vi "NMRFMTCP6test.vi"() -> ()   [LabVIEW 2013]
uses:
  <vilib>/Analysis/2dsp.llb/Power Spectrum (DBL).vi
  kleinjan/MKS/Global - Pressure & Flow.vi
  <vilib>/Analysis/NI_AALBase.lvlib
  <vilib>/Analysis/NI_AALPro.lvlib
panel:
  out "Python OK":bool=TRUE
  out "Polarization":sgl=36.423462 format="%.3f"
  out "+3.3V OK":bool=TRUE
  out "Qsub OK":bool
  out "standard error":string
  out "standard output":string
  out "return code":i32
  out "initphase":dbl=2.566 format="%#_13g"
  out "inittune":dbl=1.9 format="%#_13g"
  in  "Save Tune":bool
  in  "Tune?":bool
  out "Date / Time":string="1/31/2018 1:50:59 PM"
  in  "Stop Run":bool=TRUE
  out "He readback":bool=TRUE
  in  "Prompt?":bool
  out "He temp (K)":sgl=2.13326 format="%.3f"
  out "He press (torr)":sgl=33.89 format="%.3f"
  in  "NMR Channel Select":string(combo)="Tune2.csv"
  out "Color Box":u32(colorbox)=16775210
  out "Measurement":enum16{"TEQ", "POL", "QCV"}(ring)
  in  "VME IP Address":string="192.168.0.4"
  out "FFT Vrms":dbl[](graph)=[0.06867481296758104, 0.06857457198498951, 0.06260490220323817, 0.04579893096764441, 0.03459193119021722, 0.024334506004456635, 0.01699939743179473, 0.011320507920014591, 0.00738818639942318, 0.004922329269476129, 0.0032005220838690783, 0.002399742088009097, 0.0017369883972344268, 0.001462379050983699, 0.0012180378187000385, 0.0009973302434478017, 0.0008651345258721481, 0.0006297489865595406, 0.0005526001513740785, 0.00037281048607525053, 0.00030391613013233313, 0.00020982577489229117, 0.00011097556197799909, 9.224206231092217e-05, 6.542017012320741e-05, 9.304661554256529e-05, 5.856346737504307e-05, 7.273895027450311e-05, 7.459248680725348e-05, 2.878408363596768e-05, 6.035598396088183e-05, 1.2803091312800212e-05, 3.242558212250914e-05, 2.6299059518835237e-05, 2.8629288070241252e-05, 5.5072971721899855e-05, 6.084837494592859e-06, 1.8134519288074238e-05, 9.669082428092558e-06, 1.0358869367749575e-05, 1.018912080523636e-05, 8.60594191940927e-06, 9.591448625769922e-06, 1.1220166852002886e-05, 6.88011593273858e-06, 1.1491109330674236e-05, 1.6694054808243664e-05, 1.0324476781176234e-06, 8.726383764090988e-06, 1.0009405679331725e-05, 6.983276809422243e-06, 1.0990654268439946e-05, 6.235393540925832e-06, 1.3028318573115987e-05, 8.212929592602332e-06, 7.620469710636132e-06, 1.3517970354642288e-05, 3.1360145539364084e-06, 1.0966864774965756e-05, 1.8371644041724748e-06, 1.4366548133168728e-05, 1.8995353004426356e-05, 1.261262728619325e-05, 1.1944444533945176e-05, 6.099138601232397e-06, 1.693319713220885e-05, 1.5290407351991908e-05, 1.554922736223277e-05, 1.1123224499577624e-05, 5.543972521096801e-07, 1.2984947025426147e-05, 1.8988972689681565e-05, 1.4206861079379492e-05, 2.1083207681653224e-05, 1.6007929951300866e-05, 2.7877039602988794e-05, 1.0482172647931049e-05, 1.8537108589101367e-05, 5.604028017532567e-06, 5.635675332586378e-06, 1.0245787700958885e-05, 3.285883828179235e-06, 8.512312116457392e-06, 1.4595660468423015e-05, 3.3757230764538894e-06, 1.1434598449200437e-05, 9.009063554776636e-06, 9.09203278507544e-06, 8.614121129346514e-06, 2.7065739961170123e-06, 6.030594935431283e-06, 1.1022840446923136e-05, 3.4608859994916356e-06, 1.1678562894888675e-05, 6.324112407218391e-06, 6.1924960014341965e-06, 4.748606861354588e-06, 2.768720553267083e-06, 5.808055347668398e-06, 4.95687957388527e-06, 4.552721418323117e-06, 4.868943846160484e-06, 3.4341407516096863e-06, 5.5974628740544295e-06, 4.241367499491773e-06, 6.586740589704174e-06, 4.024549450977876e-06, 5.122947155766902e-06, 3.9773543460348965e-06, 6.5077684618683735e-06, 4.010278671524191e-06, 4.121194802615129e-06, 3.282257530443253e-06, 2.5860963363552985e-06, 9.189431625458063e-06, 7.099592745613212e-06, 5.333822391148828e-06, 5.943090011187765e-06, 4.309063888021288e-06, 3.5031630262908657e-06, 1.96922856062359e-06, 4.6071849490317016e-07, 6.351051902186674e-06, 4.122666103856541e-06, 6.469252923693759e-06, 1.8226265223917853e-06, 8.244885041838854e-06, 1.6345124528207519e-06, 4.601201303647493e-06, 8.496993206144022e-06, 3.5355491948303763e-06, 7.895706171681286e-06, 5.645936982007796e-06, 3.7385657954831592e-06, 8.727751684292659e-06, 4.869286516414961e-06, 7.81165746958526e-06, 4.667304716818145e-06, 5.081172661891545e-06, 6.686448783162224e-06, 4.00495839673786e-06, 1.1485451036657622e-05, 2.6838919673161818e-06, 1.1144088742135484e-05, 4.668724848017115e-06, 4.9955017370136556e-06, 1.6524892105897692e-06, 1.144022174967641e-06, 6.6432326246144885e-06, 4.840482493249558e-06, 1.2421741122621969e-05, 3.74322163703047e-06, 8.703797353115438e-06, 4.388068688090438e-06, 2.9175286376936667e-06, 3.3209910498661074e-06, 5.7511551959757365e-06, 3.0725434377290935e-06, 2.2189801998406774e-06, 6.073062826056792e-06, 5.407884797516531e-06, 3.323217205604381e-06, 8.478322260705957e-06, 2.4801854003522035e-06, 8.379497453356208e-06, 1.7697452972367595e-06, 7.3317561052701325e-06, 4.226726258326851e-06, 4.623660588236943e-06, 7.655373604817283e-06, 9.087980261541697e-07, 6.199940244089063e-06, 5.437223520954798e-07, 4.066597652669098e-06, 3.6919111735151345e-06, 4.291749516194073e-06, 5.610961626882009e-06, 2.5547763024940687e-06, 2.498718509567958e-06, 1.227414154389083e-05, 6.558351876350384e-06, 2.609450378482884e-06, 7.39055217848152e-06, 2.5707380987801505e-06, 5.649112772736493e-06, 5.415988675717733e-06, 5.239708070750125e-06, 2.7406394221776962e-06, 8.059224052285553e-06, 3.981707950065012e-06, 2.2827311665321965e-07, 4.762940780814428e-06, 2.2866533297097247e-06, 2.1480718211679797e-06, 8.711481544735441e-06, 4.8420425852430605e-06, 1.082893263992563e-06, 5.394159492985945e-06, 4.286252813980868e-06, 7.453130120166451e-06, 1.6277649462102944e-06, 1.6277649462102944e-06, 7.453130120166451e-06, 4.286252813980868e-06, 5.394159492985945e-06, 1.082893263992563e-06, 4.8420425852430605e-06, 8.711481544735441e-06, 2.1480718211679797e-06, 2.2866533297097247e-06, 4.762940780814428e-06, 2.2827311665321965e-07, 3.981707950065012e-06, 8.059224052285553e-06, 2.7406394221776962e-06, 5.239708070750125e-06, 5.415988675717733e-06, 5.649112772736493e-06, 2.5707380987801505e-06, 7.39055217848152e-06, 2.609450378482884e-06, 6.558351876350384e-06, 1.227414154389083e-05, 2.498718509567958e-06, 2.5547763024940687e-06, 5.610961626882009e-06, 4.291749516194073e-06, 3.6919111735151345e-06, 4.066597652669098e-06, 5.437223520954798e-07, 6.199940244089063e-06, 9.087980261541697e-07, 7.655373604817283e-06, 4.623660588236943e-06, 4.226726258326851e-06, 7.3317561052701325e-06, 1.7697452972367595e-06, 8.379497453356208e-06, 2.4801854003522035e-06, 8.478322260705957e-06, 3.323217205604381e-06, 5.407884797516531e-06, 6.073062826056792e-06, 2.2189801998406774e-06, 3.0725434377290935e-06, 5.7511551959757365e-06, 3.3209910498661074e-06, 2.9175286376936667e-06, 4.388068688090438e-06, 8.703797353115438e-06, 3.74322163703047e-06, 1.2421741122621969e-05, 4.840482493249558e-06, 6.6432326246144885e-06, 1.144022174967641e-06, 1.6524892105897692e-06, 4.9955017370136556e-06, 4.668724848017115e-06, 1.1144088742135484e-05, 2.6838919673161818e-06, 1.1485451036657622e-05, 4.00495839673786e-06, 6.686448783162224e-06, 5.081172661891545e-06, 4.667304716818145e-06, 7.81165746958526e-06, 4.869286516414961e-06, 8.727751684292659e-06, 3.7385657954831592e-06, 5.645936982007796e-06, 7.895706171681286e-06, 3.5355491948303763e-06, 8.496993206144022e-06, 4.601201303647493e-06, 1.6345124528207519e-06, 8.244885041838854e-06, 1.8226265223917853e-06, 6.469252923693759e-06, 4.122666103856541e-06, 6.351051902186674e-06, 4.6071849490317016e-07, 1.96922856062359e-06, 3.5031630262908657e-06, 4.309063888021288e-06, 5.943090011187765e-06, 5.333822391148828e-06, 7.099592745613212e-06, 9.189431625458063e-06, 2.5860963363552985e-06, 3.282257530443253e-06, 4.121194802615129e-06, 4.010278671524191e-06, 6.5077684618683735e-06, 3.9773543460348965e-06, 5.122947155766902e-06, 4.024549450977876e-06, 6.586740589704174e-06, 4.241367499491773e-06, 5.5974628740544295e-06, 3.4341407516096863e-06, 4.868943846160484e-06, 4.552721418323117e-06, 4.95687957388527e-06, 5.808055347668398e-06, 2.768720553267083e-06, 4.748606861354588e-06, 6.1924960014341965e-06, 6.324112407218391e-06, 1.1678562894888675e-05, 3.4608859994916356e-06, 1.1022840446923136e-05, 6.030594935431283e-06, 2.7065739961170123e-06, 8.614121129346514e-06, 9.09203278507544e-06, 9.009063554776636e-06, 1.1434598449200437e-05, 3.3757230764538894e-06, 1.4595660468423015e-05, 8.512312116457392e-06, 3.285883828179235e-06, 1.0245787700958885e-05, 5.635675332586378e-06, 5.604028017532567e-06, 1.8537108589101367e-05, 1.0482172647931049e-05, 2.7877039602988794e-05, 1.6007929951300866e-05, 2.1083207681653224e-05, 1.4206861079379492e-05, 1.8988972689681565e-05, 1.2984947025426147e-05, 5.543972521096801e-07, 1.1123224499577624e-05, 1.554922736223277e-05, 1.5290407351991908e-05, 1.693319713220885e-05, 6.099138601232397e-06, 1.1944444533945176e-05, 1.261262728619325e-05, 1.8995353004426356e-05, 1.4366548133168728e-05, 1.8371644041724748e-06, 1.0966864774965756e-05, 3.1360145539364084e-06, 1.3517970354642288e-05, 7.620469710636132e-06, 8.212929592602332e-06, 1.3028318573115987e-05, 6.235393540925832e-06, 1.0990654268439946e-05, 6.983276809422243e-06, 1.0009405679331725e-05, 8.726383764090988e-06, 1.0324476781176234e-06, 1.6694054808243664e-05, 1.1491109330674236e-05, 6.88011593273858e-06, 1.1220166852002886e-05, 9.591448625769922e-06, 8.60594191940927e-06, 1.018912080523636e-05, 1.0358869367749575e-05, 9.669082428092558e-06, 1.8134519288074238e-05, 6.084837494592859e-06, 5.5072971721899855e-05, 2.8629288070241252e-05, 2.6299059518835237e-05, 3.242558212250914e-05, 1.2803091312800212e-05, 6.035598396088183e-05, 2.878408363596768e-05, 7.459248680725348e-05, 7.273895027450311e-05, 5.856346737504307e-05, 9.304661554256529e-05, 6.542017012320741e-05, 9.224206231092217e-05, 0.00011097556197799909, 0.00020982577489229117, 0.00030391613013233313, 0.00037281048607525053, 0.0005526001513740785, 0.0006297489865595406, 0.0008651345258721481, 0.0009973302434478017, 0.0012180378187000385, 0.001462379050983699, 0.0017369883972344268, 0.002399742088009097, 0.0032005220838690783, 0.004922329269476129, 0.00738818639942318, 0.011320507920014591, 0.01699939743179473, 0.024334506004456635, 0.03459193119021722, 0.04579893096764441, 0.06260490220323817, 0.06857457198498951]
  out "Raw NMR Graph / Ave":cluster{dbl, "Step Width (MHz)":dbl, dbl[][]}(graph)={212.6, "Step Width (MHz)"=0.002, [[0.0092, 0.0092, 0.0092, 0.009, 0.0087, 0.0085, 0.0082, 0.0078, 0.0075, 0.0072, 0.0069, 0.0066, 0.0061, 0.006, 0.0058, 0.0055, 0.0052, 0.005, 0.0047, 0.0044, 0.0043, 0.0041, 0.0041, 0.0037, 0.0037, 0.0034, 0.0032, 0.0029, 0.0024, 0.0021, 0.0017, 0.0015, 0.0012, 0.0009, 0.0008, 0.0008, 0.0006, 0.0005, 0.0003, 0.0003, -0.0, -0.0002, -0.0005, -0.0006, -0.0009, -0.0011, -0.0014, -0.0017, -0.0018, -0.002, -0.0023, -0.0026, -0.0026, -0.0027, -0.0027, -0.0031, -0.0029, -0.0032, -0.0032, -0.0032, -0.0034, -0.0037, -0.0037, -0.0041, -0.0043, -0.0044, -0.0046, -0.0047, -0.0047, -0.0047, -0.0049, -0.0049, -0.005, -0.0049, -0.005, -0.0052, -0.0055, -0.0055, -0.0056, -0.0056, -0.0056, -0.0058, -0.006, -0.0061, -0.0061, -0.0063, -0.0063, -0.0064, -0.0064, -0.0064, -0.0064, -0.0063, -0.0061, -0.0061, -0.0061, -0.0061, -0.0061, -0.0061, -0.0061, -0.0061, -0.0063, -0.0063, -0.0061, -0.006, -0.006, -0.0056, -0.0053, -0.0052, -0.005, -0.0049, -0.0047, -0.0044, -0.0043, -0.0041, -0.0038, -0.0037, -0.0034, -0.0031, -0.0029, -0.0026, -0.0024, -0.0021, -0.0018, -0.0015, -0.0009, -0.0006, -0.0, 0.0003, 0.0009, 0.0015, 0.002, 0.0026, 0.0031, 0.0035, 0.0041, 0.0047, 0.0052, 0.0058, 0.0066, 0.0073, 0.0082, 0.0092, 0.0099, 0.011, 0.0119, 0.013, 0.014, 0.0151, 0.016, 0.0172, 0.0186, 0.0198, 0.0211, 0.0223, 0.0237, 0.0253, 0.027, 0.029, 0.0308, 0.033, 0.0352, 0.0378, 0.0403, 0.043, 0.0461, 0.049, 0.0522, 0.0555, 0.0592, 0.0632, 0.0674, 0.0722, 0.0771, 0.0822, 0.0879, 0.094, 0.1006, 0.1074, 0.1144, 0.1224, 0.1309, 0.1401, 0.1495, 0.1593, 0.1697, 0.1808, 0.1926, 0.2049, 0.2179, 0.231, 0.2454, 0.2605, 0.2759, 0.2922, 0.3087, 0.3261, 0.3433, 0.3609, 0.3789, 0.3967, 0.4143, 0.4314, 0.4485, 0.4655, 0.4817, 0.4973, 0.5115, 0.5258, 0.5396, 0.5525, 0.5644, 0.5754, 0.5856, 0.5954, 0.6039, 0.6108, 0.6163, 0.6203, 0.6227, 0.623, 0.6213, 0.6169, 0.6105, 0.6018, 0.591, 0.5774, 0.5606, 0.5417, 0.5203, 0.497, 0.4721, 0.4446, 0.4161, 0.3874, 0.3583, 0.3307, 0.304, 0.2774, 0.2525, 0.2295, 0.2086, 0.1898, 0.1729, 0.1567, 0.1419, 0.1286, 0.1166, 0.1057, 0.0954, 0.0859, 0.0775, 0.0699, 0.0627, 0.0562, 0.0502, 0.0447, 0.0397, 0.0352, 0.0308, 0.027, 0.0237, 0.0204, 0.0177, 0.015, 0.0125, 0.0104, 0.0082, 0.0066, 0.0047, 0.0031, 0.0015, -0.0, -0.0014, -0.0027, -0.0041, -0.0052, -0.0064, -0.0073, -0.0082, -0.0093, -0.0101, -0.0108, -0.0114, -0.0121, -0.0127, -0.0131, -0.0134, -0.0139, -0.0143, -0.0146, -0.0151, -0.0157, -0.0163, -0.0166, -0.0169, -0.0172, -0.0172, -0.0175, -0.0175, -0.0177, -0.0175, -0.0177, -0.0175, -0.0177, -0.0177, -0.0177, -0.0179, -0.0179, -0.0179, -0.0179, -0.0179, -0.0179, -0.0179, -0.0179, -0.0177, -0.0179, -0.0175, -0.0175, -0.0172, -0.0171, -0.0168, -0.0165, -0.0163, -0.016, -0.016, -0.0159, -0.0159, -0.0156, -0.0154, -0.0154, -0.0151, -0.0148, -0.0145, -0.0142, -0.0139, -0.0137, -0.0134, -0.0133, -0.013, -0.0128, -0.0125, -0.0124, -0.0119, -0.0117, -0.0114, -0.011, -0.0108, -0.0107, -0.0104, -0.0104, -0.0099, -0.0098, -0.0096, -0.0092, -0.0087, -0.0084, -0.0079, -0.0076, -0.0073, -0.007, -0.0069, -0.0067, -0.0064, -0.0061, -0.0058, -0.0056, -0.0052, -0.0049, -0.0046, -0.0043, -0.0038, -0.0037, -0.0031, -0.0027, -0.0023, -0.002, -0.0015, -0.0011, -0.0008, -0.0005, -0.0002, -0.0, 0.0002, 0.0006, 0.0008, 0.0012, 0.0015, 0.002, 0.0026, 0.0031, 0.0037, 0.004, 0.0044, 0.0047, 0.0049, 0.0053, 0.0056, 0.0058, 0.0061, 0.0063, 0.0066], [0.0, 0.0, 0.0, 0.0, 0.0, 0.0, 0.0, 0.0, 0.0, 0.0, 0.0, 0.0, 0.0, 0.0, 0.0, 0.0, 0.0, 0.0, 0.0, 0.0, 0.0, 0.0, 0.0, 0.0, 0.0, 0.0, 0.0, 0.0, 0.0, 0.0, 0.0, 0.0, 0.0, 0.0, 0.0, 0.0, 0.0, 0.0, 0.0, 0.0, 0.0, 0.0, 0.0, 0.0, 0.0, 0.0, 0.0, 0.0, 0.0, 0.0, 0.0, 0.0, 0.0, 0.0, 0.0, 0.0, 0.0, 0.0, 0.0, 0.0, 0.0, 0.0, 0.0, 0.0, 0.0, 0.0, 0.0, 0.0, 0.0, 0.0, 0.0, 0.0, 0.0, 0.0, 0.0, 0.0, 0.0, 0.0, 0.0, 0.0, 0.0, 0.0, 0.0, 0.0, 0.0, 0.0, 0.0, 0.0, 0.0, 0.0, 0.0, 0.0, 0.0, 0.0, 0.0, 0.0, 0.0, 0.0, 0.0, 0.0, 0.0, 0.0, 0.0, 0.0, 0.0, 0.0, 0.0, 0.0, 0.0, 0.0, 0.0, 0.0, 0.0, 0.0, 0.0, 0.0, 0.0, 0.0, 0.0, 0.0, 0.0, 0.0, 0.0, 0.0, 0.0, 0.0, 0.0, 0.0, 0.0, 0.0, 0.0, 0.0, 0.0, 0.0, 0.0, 0.0, 0.0, 0.0, 0.0, 0.0, 0.0, 0.0, 0.0, 0.0, 0.0, 0.0, 0.0, 0.0, 0.0, 0.0, 0.0, 0.0, 0.0, 0.0, 0.0, 0.0, 0.0, 0.0, 0.0, 0.0, 0.0, 0.0, 0.0, 0.0, 0.0, 0.0, 0.0, 0.0, 0.0, 0.0, 0.0, 0.0, 0.0, 0.0, 0.0, 0.0, 0.0, 0.0, 0.0, 0.0, 0.0, 0.0, 0.0, 0.0, 0.0, 0.0, 0.0, 0.0, 0.0, 0.0, 0.0, 0.0, 0.0, 0.0, 0.0, 0.0, 0.0, 0.0, 0.0, 0.0, 0.0, 0.0, 0.0, 0.0, 0.0, 0.0, 0.0, 0.0, 0.0, 0.0, 0.0, 0.0, 0.0, 0.0, 0.0, 0.0, 0.0, 0.0, 0.0, 0.0, 0.0, 0.0, 0.0, 0.0, 0.0, 0.0, 0.0, 0.0, 0.0, 0.0, 0.0, 0.0, 0.0, 0.0, 0.0, 0.0, 0.0, 0.0, 0.0, 0.0, 0.0, 0.0, 0.0, 0.0, 0.0, 0.0, 0.0, 0.0, 0.0, 0.0, 0.0, 0.0, 0.0, 0.0, 0.0, 0.0, 0.0, 0.0, 0.0, 0.0, 0.0, 0.0, 0.0, 0.0, 0.0, 0.0, 0.0, 0.0, 0.0, 0.0, 0.0, 0.0, 0.0, 0.0, 0.0, 0.0, 0.0, 0.0, 0.0, 0.0, 0.0, 0.0, 0.0, 0.0, 0.0, 0.0, 0.0, 0.0, 0.0, 0.0, 0.0, 0.0, 0.0, 0.0, 0.0, 0.0, 0.0, 0.0, 0.0, 0.0, 0.0, 0.0, 0.0, 0.0, 0.0, 0.0, 0.0, 0.0, 0.0, 0.0, 0.0, 0.0, 0.0, 0.0, 0.0, 0.0, 0.0, 0.0, 0.0, 0.0, 0.0, 0.0, 0.0, 0.0, 0.0, 0.0, 0.0, 0.0, 0.0, 0.0, 0.0, 0.0, 0.0, 0.0, 0.0, 0.0, 0.0, 0.0, 0.0, 0.0, 0.0, 0.0, 0.0, 0.0, 0.0, 0.0, 0.0, 0.0, 0.0, 0.0, 0.0, 0.0, 0.0, 0.0, 0.0, 0.0, 0.0, 0.0, 0.0, 0.0, 0.0, 0.0, 0.0, 0.0, 0.0, 0.0, 0.0, 0.0, 0.0, 0.0, 0.0, 0.0, 0.0, 0.0, 0.0, 0.0, 0.0, 0.0, 0.0, 0.0, 0.0, 0.0, 0.0, 0.0, 0.0, 0.0, 0.0, 0.0, 0.0, 0.0, 0.0, 0.0, 0.0, 0.0, 0.0, 0.0, 0.0, 0.0, 0.0, 0.0, 0.0], [0.0, 0.0, 0.0, 0.0, 0.0, 0.0, 0.0, 0.0, 0.0, 0.0, 0.0, 0.0, 0.0, 0.0, 0.0, 0.0, 0.0, 0.0, 0.0, 0.0, 0.0, 0.0, 0.0, 0.0, 0.0, 0.0, 0.0006, 0.0006, 0.0004, 0.0003, 0.0003, 0.0003, 0.0001, 0.0, -0.0001, -0.0001, -0.0001, -0.0001, -0.0001, -0.0002, -0.0002, -0.0002, -0.0003, -0.0003, -0.0003, -0.0002, -0.0003, -0.0002, -0.0002, -0.0001, -0.0002, -0.0002, -0.0002, -0.0002, -0.0002, -0.0003, -0.0003, -0.0002, -0.0002, -0.0001, -0.0002, -0.0001, -0.0001, -0.0001, -0.0001, -0.0001, 0.0001, 0.0001, 0.0002, 0.0003, 0.0004, 0.0005, 0.0005, 0.0006, 0.0007, 0.0007, 0.0007, 0.0008, 0.0008, 0.001, 0.0011, 0.0012, 0.0013, 0.0015, 0.0016, 0.0016, 0.0018, 0.0019, 0.0021, 0.0022, 0.0023, 0.0025, 0.0028, 0.0029, 0.0031, 0.0033, 0.0035, 0.0037, 0.0039, 0.0041, 0.0042, 0.0044, 0.0047, 0.005, 0.0053, 0.0056, 0.006, 0.0062, 0.0065, 0.0067, 0.0072, 0.0074, 0.0077, 0.0081, 0.0086, 0.009, 0.0093, 0.0099, 0.0103, 0.0108, 0.0112, 0.0116, 0.012, 0.0125, 0.0131, 0.0136, 0.0141, 0.0147, 0.0154, 0.016, 0.0166, 0.0173, 0.0179, 0.0186, 0.0193, 0.0201, 0.0208, 0.0217, 0.0226, 0.0235, 0.0244, 0.0254, 0.0263, 0.0272, 0.0283, 0.0293, 0.0305, 0.0316, 0.0328, 0.0341, 0.0355, 0.037, 0.0385, 0.0399, 0.0415, 0.0433, 0.0452, 0.0471, 0.0491, 0.0514, 0.0537, 0.0562, 0.0588, 0.0616, 0.0646, 0.0678, 0.0712, 0.0748, 0.0786, 0.0828, 0.0872, 0.092, 0.097, 0.1023, 0.108, 0.1141, 0.1208, 0.1275, 0.1347, 0.1427, 0.1512, 0.1606, 0.17, 0.1796, 0.1902, 0.2015, 0.2135, 0.2259, 0.2388, 0.2523, 0.2668, 0.282, 0.2974, 0.3138, 0.3302, 0.3475, 0.365, 0.3826, 0.4006, 0.4185, 0.4362, 0.4535, 0.4706, 0.4876, 0.504, 0.5195, 0.5338, 0.5482, 0.5621, 0.5751, 0.5871, 0.598, 0.6084, 0.6181, 0.6266, 0.6335, 0.639, 0.643, 0.6453, 0.6458, 0.6438, 0.6396, 0.6333, 0.6247, 0.614, 0.6005, 0.584, 0.565, 0.5435, 0.5202, 0.4953, 0.4677, 0.4392, 0.4106, 0.3814, 0.3539, 0.3271, 0.3006, 0.2759, 0.2529, 0.2321, 0.2135, 0.1966, 0.1805, 0.1657, 0.1524, 0.1404, 0.1295, 0.1191, 0.1095, 0.101, 0.0931, 0.0862, 0.0795, 0.0733, 0.068, 0.0629, 0.0585, 0.0542, 0.0505, 0.0471, 0.0439, 0.0411, 0.0383, 0.0358, 0.0335, 0.0313, 0.0293, 0.0274, 0.0257, 0.024, 0.0225, 0.0212, 0.0198, 0.0185, 0.0174, 0.0163, 0.0152, 0.0143, 0.0134, 0.0125, 0.0116, 0.0108, 0.0101, 0.0094, 0.0088, 0.0083, 0.0077, 0.0072, 0.0067, 0.0062, 0.0056, 0.0053, 0.0048, 0.0044, 0.004, 0.0037, 0.0035, 0.0033, 0.003, 0.0028, 0.0025, 0.0023, 0.002, 0.0018, 0.0016, 0.0015, 0.0013, 0.0012, 0.0011, 0.001, 0.0009, 0.0008, 0.0007, 0.0006, 0.0004, 0.0004, 0.0003, 0.0003, 0.0003, 0.0002, 0.0003, 0.0002, 0.0002, 0.0002, 0.0001, 0.0001, 0.0, -0.0, -0.0, -0.0, 0.0, 0.0, 0.0001, 0.0001, 0.0, 0.0001, -0.0001, -0.0001, -0.0001, -0.0002, -0.0001, -0.0, -0.0, 0.0, 0.0, 0.0001, 0.0, 0.0001, 0.0, -0.0, -0.0, -0.0001, -0.0, 0.0001, 0.0001, 0.0001, 0.0, 0.0001, 0.0001, -0.0, -0.0, -0.0001, -0.0, 0.0, 0.0, 0.0001, 0.0001, 0.0, 0.0, 0.0001, -0.0, -0.0, -0.0001, -0.0001, 0.0, 0.0, 0.0, 0.0, 0.0, 0.0, 0.0, 0.0, 0.0, 0.0, 0.0, 0.0, 0.0, 0.0, 0.0, 0.0, 0.0, 0.0, 0.0, 0.0, 0.0, 0.0, 0.0, 0.0, 0.0, 0.0]]}
  in  "R&S GPIB Addr (28)":refnum<visa-resource-name>="GPIB0::28::INSTR"
  out "Pedestal (V)":dbl=-0.005459583333333334 format="%_2g"
  in  "Open Global Panel":bool
  out "Peak center (MHz)":sgl=213.038 format="%.3f"
  out "Telnet error out":errorcluster
  out "+3.3V supply":dbl=3.279 format="%_4g"
  out "Temp (C)":dbl=28.0 format="%_4g"
  out "RF level OK":bool=TRUE
  out "Polarization %":sgl=36.423462 format="%.3e"
  out "# Good Spectra":i32=494
  out "Pedestal volts OK":bool=TRUE
  out "Sweep #":i32=1
  out "1st Sweep":bool
  out "ADC volts OK":bool=TRUE
  out "Peak Height Distribution":cluster{"Y":dbl[], "Y":dbl[]}[](graph)=[{"Y"=[1.4880254648797504, 1.4904694004799532, 1.492913336080156, 1.495357271680359, 1.4978012072805618, 1.5002451428807646, 1.5026890784809674, 1.5051330140811703, 1.5075769496813731, 1.510020885281576, 1.5124648208817788, 1.5149087564819816, 1.5173526920821847, 1.5197966276823875, 1.5222405632825904, 1.5246844988827932, 1.527128434482996, 1.529572370083199, 1.5320163056834017, 1.5344602412836046, 1.5369041768838074, 1.5393481124840103, 1.541792048084213, 1.544235983684416, 1.5466799192846188, 1.5491238548848218, 1.5515677904850247, 1.5540117260852275, 1.5564556616854304, 1.5588995972856332, 1.561343532885836, 1.563787468486039, 1.5662314040862417, 1.5686753396864446, 1.5711192752866474, 1.5735632108868502, 1.576007146487053, 1.5784510820872562, 1.580895017687459, 1.5833389532876618, 1.5857828888878647, 1.5882268244880675, 1.5906707600882704, 1.5931146956884732, 1.595558631288676, 1.5980025668888789, 1.6004465024890817, 1.6028904380892846, 1.6053343736894874, 1.6077783092896902, 1.6102222448898933, 1.6126661804900961, 1.615110116090299, 1.6175540516905018, 1.6199979872907047, 1.6224419228909075, 1.6248858584911103, 1.6273297940913132, 1.629773729691516, 1.6322176652917189, 1.6346616008919217, 1.6371055364921245, 1.6395494720923276, 1.6419934076925304, 1.6444373432927333, 1.6468812788929361, 1.649325214493139, 1.6517691500933418, 1.6542130856935446, 1.6566570212937475, 1.6591009568939503, 1.6615448924941532, 1.663988828094356, 1.6664327636945588, 1.6688766992947617, 1.6713206348949647, 1.6737645704951676, 1.6762085060953704, 1.6786524416955733, 1.681096377295776, 1.683540312895979, 1.6859842484961818, 1.6884281840963846, 1.6908721196965875, 1.6933160552967903, 1.6957599908969931, 1.698203926497196, 1.700647862097399, 1.7030917976976019, 1.7055357332978047, 1.7079796688980076, 1.7104236044982104, 1.7128675400984132, 1.715311475698616, 1.717755411298819, 1.7201993468990218, 1.7226432824992246, 1.7250872180994274, 1.7275311536996303, 1.7299750892998331], "Y"=[3.0, 0.0, 0.0, 2.0, 1.0, 1.0, 0.0, 0.0, 2.0, 0.0, 2.0, 1.0, 2.0, 4.0, 2.0, 2.0, 0.0, 2.0, 2.0, 1.0, 5.0, 6.0, 7.0, 4.0, 5.0, 7.0, 3.0, 5.0, 5.0, 4.0, 5.0, 4.0, 7.0, 14.0, 7.0, 9.0, 12.0, 12.0, 8.0, 3.0, 5.0, 7.0, 6.0, 7.0, 8.0, 11.0, 7.0, 15.0, 12.0, 15.0, 15.0, 11.0, 8.0, 6.0, 11.0, 5.0, 6.0, 11.0, 14.0, 5.0, 6.0, 12.0, 9.0, 9.0, 3.0, 8.0, 13.0, 5.0, 6.0, 4.0, 10.0, 3.0, 5.0, 2.0, 6.0, 4.0, 5.0, 1.0, 4.0, 6.0, 3.0, 2.0, 0.0, 3.0, 4.0, 2.0, 2.0, 0.0, 2.0, 0.0, 4.0, 1.0, 2.0, 2.0, 0.0, 0.0, 0.0, 1.0, 0.0, 1.0]}]
  out "S/N":dbl=34.03525335839496 format="%_3g"
  out "Polarization %":dbl=1.6080975834470894 format="%_4g"
  out "Pedestal Diff (V)":sgl=-0.008144166 format="%.4f"
  out "Peak amp (mV)":sgl=351.93738 format="%.4f"
  out "SMT error out":errorcluster
  out "Pol sdev":dbl=47.24799802468473 format="%.3f"
  # "E1039 NMR Panel"
  # "Results"
  # "A\nv\ne\nr\na\ng\ne\ns"
  # "S\nw\ne\ne\np"
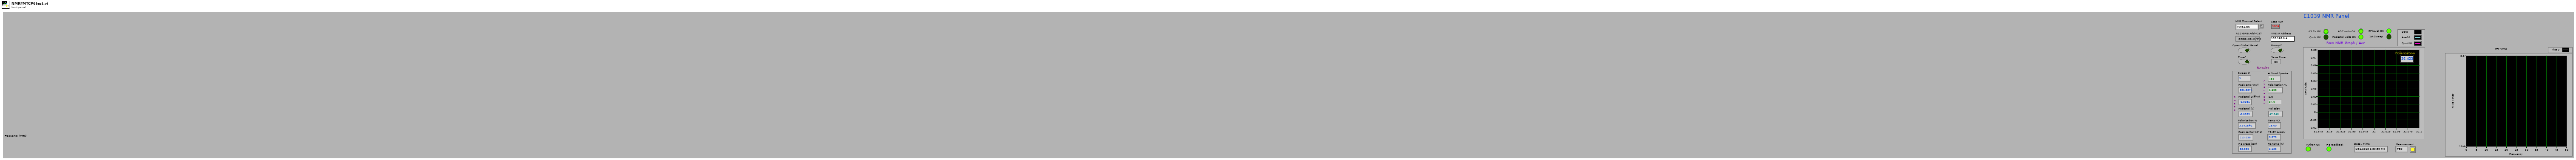
[diagram p1: front panel]
types:
  T1 = enum32{"Invalid", "Standard", "Closed", "Hidden", "Minimized", "Maximized"}
  T2 = enum32{"Bad", "Idle", "Run top level", "Running"}
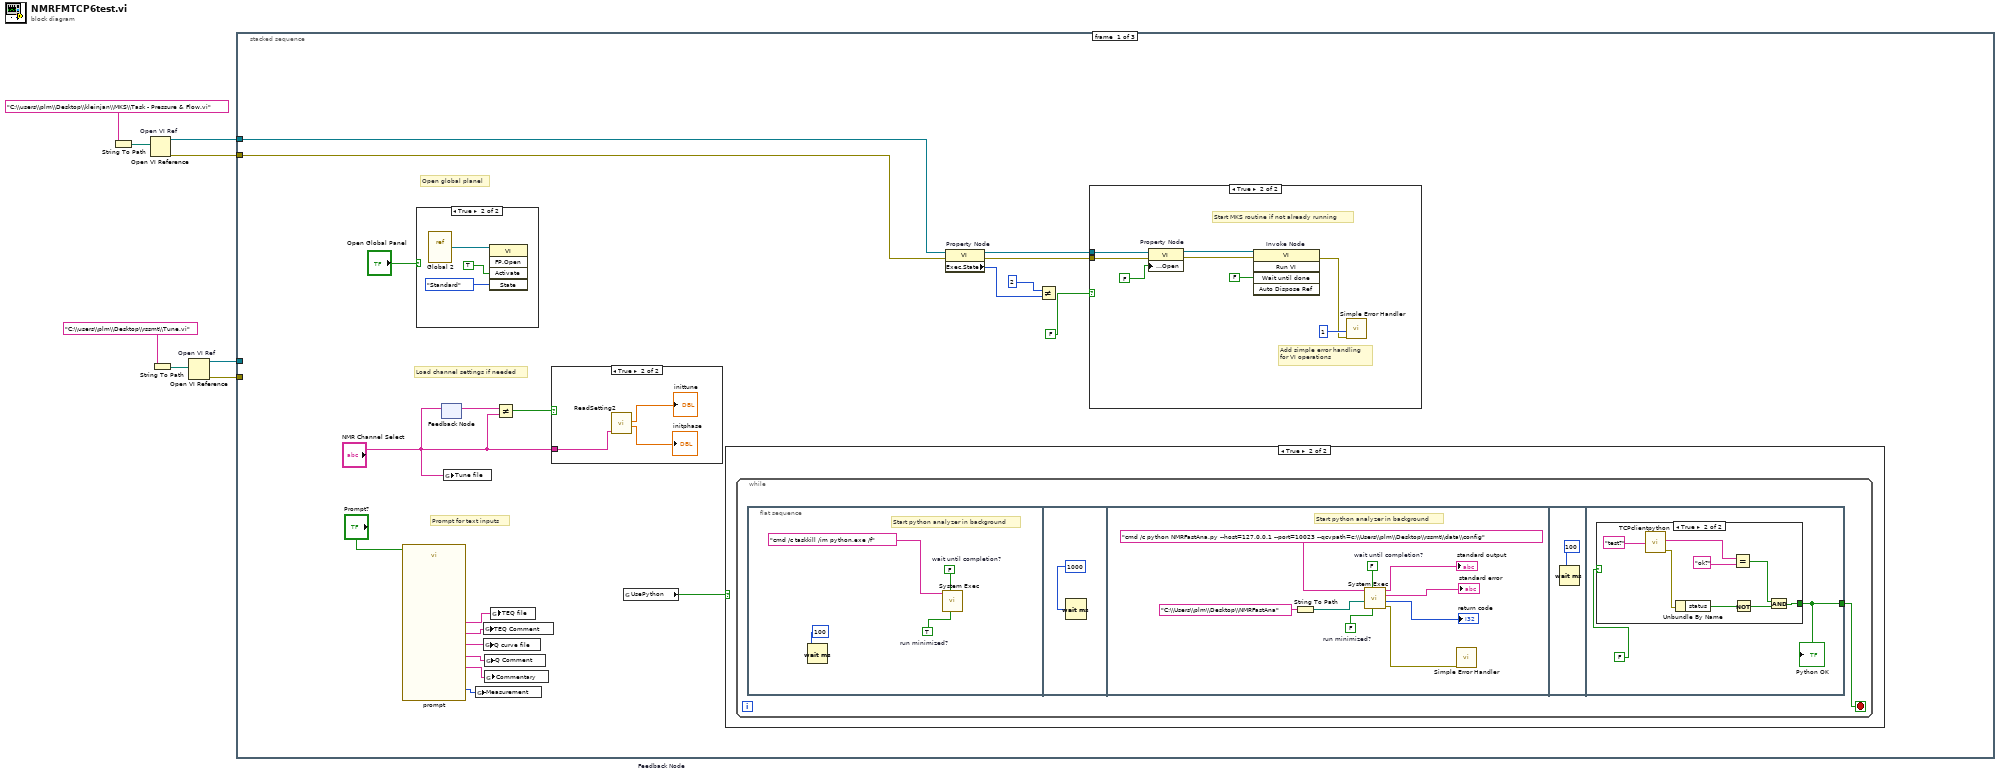
[diagram p0: block diagram]
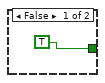
[diagram p3: hidden frame]
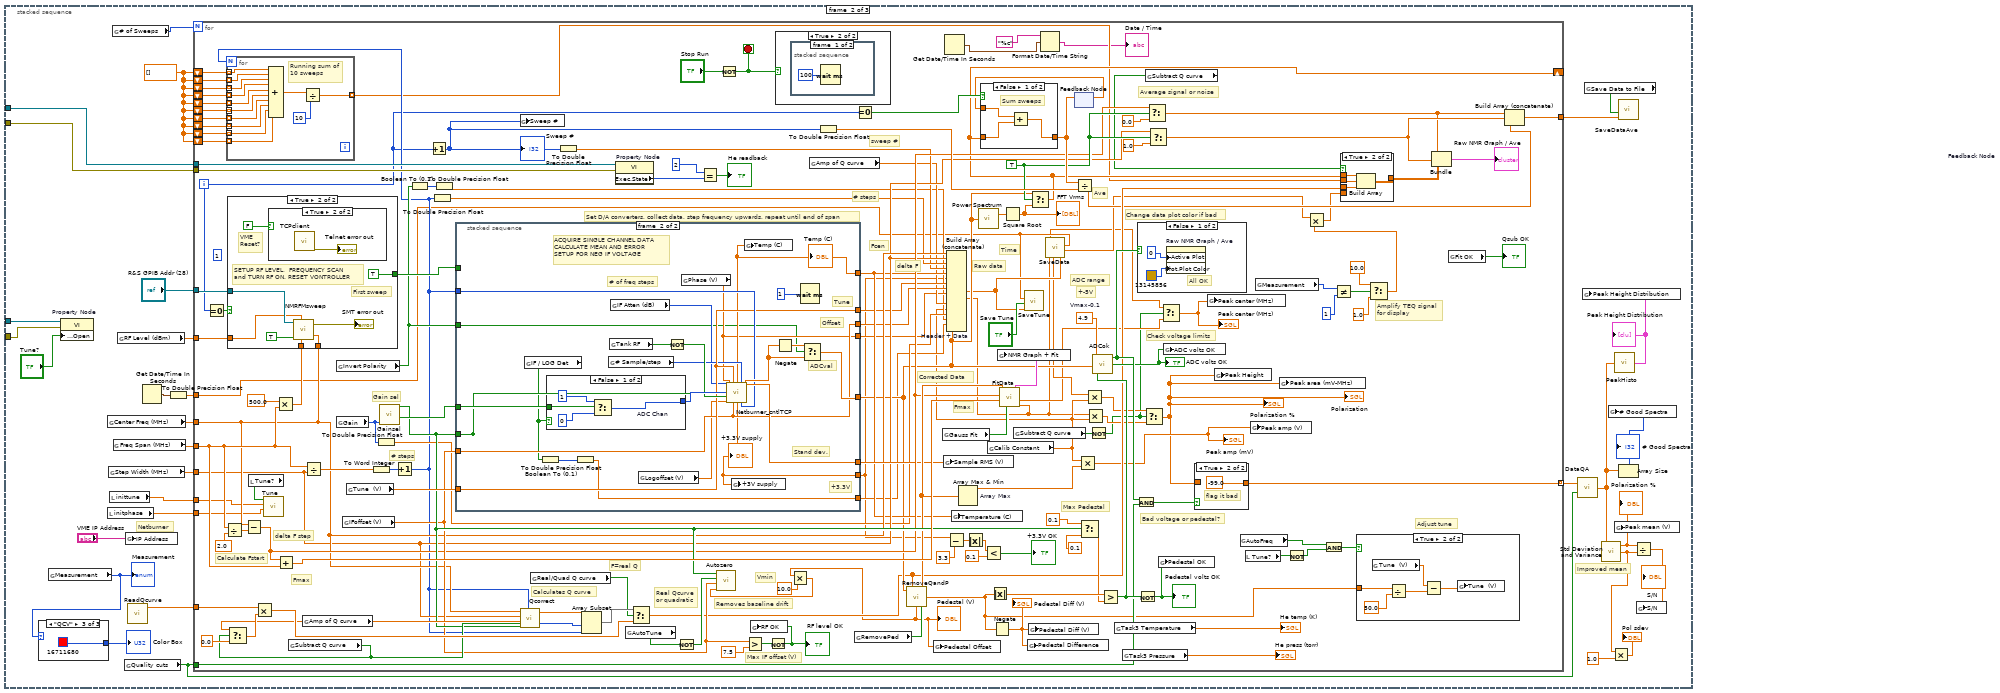
[diagram p7: hidden frame]
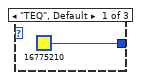
[diagram p8: hidden frame]
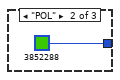
[diagram p9: hidden frame]
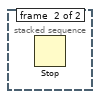
[diagram p12: hidden frame]
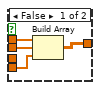
[diagram p13: hidden frame]
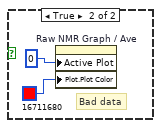
[diagram p15: hidden frame]
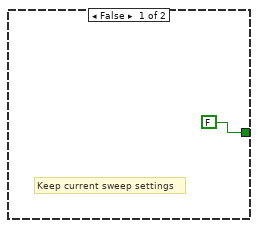
[diagram p17: hidden frame]
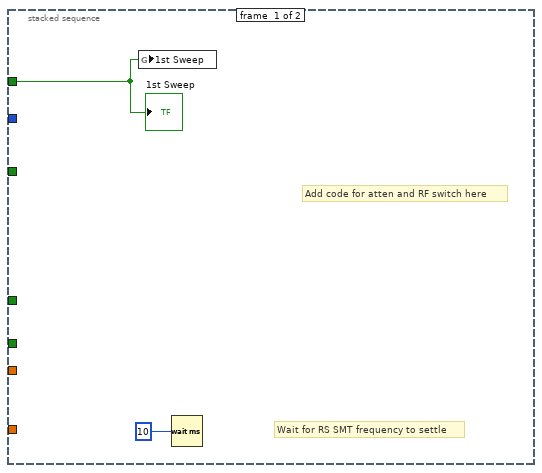
[diagram p19: hidden frame]
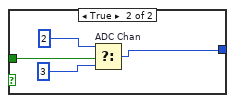
[diagram p20: hidden frame]
diagram:
  n1 = String To Path(string="C:\\users\\plm\\Desktop\\kleinjan\\MKS\\Task - Pressure & Flow.vi") -> (path=w8:path)
  n2 = Open VI Reference "Open VI Ref"(vi path=w8) -> (vi reference=w5:refnum<vi>, error out=w6:errorcluster)  [unwired: 5 in]
  n3 = String To Path(string="C:\\users\\plm\\Desktop\\rssmt\\Tune.vi") -> (path=w4:path)
  n4 = Open VI Reference "Open VI Ref"(vi path=w4) -> (vi reference=w2:refnum<vi>, error out=w1:errorcluster)  [unwired: 5 in]
  n5 = stacked-sequence {
    tunnel: w5 -> [w12 w76 w337]
    tunnel: w6 -> [w11 w75 w336]
    tunnel: w2 -> [_ w69 _]
    tunnel: w1 -> [_ w73 _]
    frame #0 {
      # "Prompt for text inputs"
      # "Load channel settings if needed"
      # "Open global planel"
      n6 = call "prompt.vi"("Enable"="Prompt?") -> ("Measurement"=w25:enum16{"TEQ", "POL", "QCV"}, "Run comment"=w24:string, "Q curve comment"=w23:string, "Q curve file"=w22:string, "TE Comment"=w21:string, "TE peak file"=w20:string)  [unwired: 11 in, 2 out]
      n7 = case shown="True" "Open Global Panel" {
        frame False {
        }
        frame True {
          n8 = vi-ref "Global 2.vi"() -> (w68:refnum<vi>)
          n9 = invoke class="VI" method="FP.Open"(reference=w68, "Activate"=TRUE, "State"=T1."Standard") -> ()  [unwired: 2 in, 5 out]
        }
      }
      n10 = feedback #1 "Feedback Node"() -> (w19:string)  [unwired: 1 in]
      n11 = feedback-in #1("NMR Channel Select") -> ()
      n12 = global write "Global 2.vi" "Tune file"("NMR Channel Select") -> ()
      n13 = global write "Global 2.vi" "Measurement"(w25) -> ()
      n14 = global write "Global 2.vi" "TEQ Comment"(w21) -> ()
      n15 = global write "Global 2.vi" "Q curve file"(w22) -> ()
      n16 = global write "Global 2.vi" "Q Comment"(w23) -> ()
      n17 = global write "Global 2.vi" "Commentary"(w24) -> ()
      n18 = global write "Global 2.vi" "TEQ file"(w20) -> ()
      n19 = Not Equal?(x=w19, y="NMR Channel Select") -> (x != y?=w18:bool)
      n20 = case shown="True" w18 {
        tunnel: "NMR Channel Select" -> [_ w65]
        frame False {
        }
        frame True {
          n21 = call "ReadSetting2.vi"("Data Filename"=w65) -> ("Phase"=→"initphase":dbl, "Tune"=→"inittune":dbl)  [unwired: 1 out]
        }
      }
      n22 = global read "Global 2.vi" "UsePython"() -> (w9:bool)
      n23 = case shown="True" w9 {
        frame False {
        }
        frame True {
          n24 = while {
            stop <- w28 stop-if-true
            n25 = flat-sequence {
              tunnel: [w45] -> w28
              frame #0 {
                w29 = TRUE  # run minimized?
                w30 = FALSE  # wait until completion?
                # "Start python analyzer in background"
                n26 = Wait (ms)(milliseconds to wait=100) -> ()  [unwired: 1 out]
                n27 = call <vilib>:"System Exec.vi"("run minimized? (F)"=w29, "wait until completion? (T)"=w30, "command line"="cmd /c taskkill /im python.exe /f") -> ()  [unwired: 5 in, 4 out]
              }
              frame #1 {
                n28 = Wait (ms)(milliseconds to wait=1000) -> ()  [unwired: 1 out]
              }
              frame #2 {
                w40 = FALSE  # run minimized?
                w41 = FALSE  # wait until completion?
                # "Start python analyzer in background"
                n29 = String To Path(string="C:\\Users\\plm\\Desktop\\NMRFastAna") -> (path=w35:path)
                n30 = call <vilib>:"System Exec.vi"("run minimized? (F)"=w40, "wait until completion? (T)"=w41, "working directory"=w35, "command line"="cmd /c python NMRFastAna.py --host=127.0.0.1 --port=10023 --qcvpath=c:\\Users\\plm\\Desktop\\rssmt\\data\\config") -> ("error out"=w36:errorcluster, "return code"=→"return code":i32, "standard error"=→"standard error":string, "standard output"=→"standard output":string)  [unwired: 4 in]
                n31 = call <vilib>:"Simple Error Handler.vi"("error in (no error)"=w36) -> ()  [unwired: 1 in, 8 out]
              }
              frame #3 {
                n32 = Wait (ms)(milliseconds to wait=100) -> ()  [unwired: 1 out]
              }
              frame #4 {
                n33 = case shown="True" FALSE {
                  tunnel: [TRUE w50] -> w45
                  frame False {
                  }
                  frame True {
                    n34 = call "TCPclientpython.vi"("Input Command"="test?") -> ("Telnet error"=w48:errorcluster, "Command and Results"=w53:string)  [unwired: 4 in, 1 out]
                    n35 = Unbundle By Name(w48) -> ("status"=w47:bool)
                    n36 = Equal?(x=w53, y="ok?") -> (x = y?=w51:bool)
                    n37 = Not(x=w47) -> (.not. x?=w49:bool)
                    n38 = And(x=w51, y=w49) -> (x .and. y?=w50:bool)
                  }
                }
                "Python OK" <- w45
              }
            }
          }
        }
      }
      n39 = property on="Property Node" class="VI"(reference=w12, error in=w11) -> (reference out=w14:refnum<vi>, error out=w13:errorcluster, "Exec.State"=w15:T2)
      n40 = Not Equal?(x=2, y=w15) -> ()  [unwired: 1 out]
      n41 = case shown="True" FALSE {
        tunnel: w14 -> [_ w59]
        tunnel: w13 -> [_ w58]
        frame False {
        }
        frame True {
          # "Start MKS routine if not already running"
          # "Add simple error handling\nfor VI operations"
          n42 = property on="Property Node" class="VI"(reference=w59, error in=w58, "Front Panel Window:Open"=FALSE ("Front Panel.Open")) -> (reference out=w57:refnum<vi>, error out=w56:errorcluster)
          n43 = invoke on="Invoke Node" class="VI" method="Run VI"(reference=w57, error in=w56, "Wait until done"=FALSE) -> (error out=w60:errorcluster)  [unwired: 2 in, 4 out]
          n44 = call <vilib>:"Simple Error Handler.vi"("type of dialog (OK msg:1)"=1, "error in (no error)"=w60) -> ()  [unwired: 3 in, 5 out]
        }
      }
    }
    frame #1 {
      w74 = dbl[] []
      # "Netburner"
      # "Improved mean"
      n45 = global read "Global 2.vi" "Measurement"() -> (w78:enum16{"TEQ", "POL", "QCV"})
      "Measurement" <- w78
      n46 = case shown="\"QCV\"" w78 {
        tunnel: [u32 16775210 ("Color Box 2") u32 3852288 ("Color Box 2") u32 16711680 ("Color Box 2")] -> w77
        frame "TEQ", Default {
        }
        frame "POL" {
        }
        frame "QCV" {
        }
      }
      "Color Box" <- w77
      n47 = property on="Property Node" class="VI"(reference=w69, error in=w73, "Front Panel Window:Open"="Tune?") -> ()  [unwired: 2 out]
      n48 = global read "Global 2.vi" "Center Freq (MHz)"() -> (w95:dbl)
      n49 = local read "initphase"() -> (w70:dbl)
      n50 = global read "Global 2.vi" "Step Width (MHz)"() -> (w93:dbl)
      n51 = local read "inittune"() -> (w71:dbl)
      n52 = global read "Global 2.vi" "# of Sweeps"() -> (w97:i32)
      n53 = global read "Global 2.vi" "Freq Span (MHz)"() -> (w94:dbl)
      n54 = global read "Global 2.vi" "RF Level (dBm)"() -> (w96:dbl)
      n55 = global read "Global 2.vi" "Quality cuts"() -> (w92:bool)
      n56 = global write "Global 2.vi" "IP Address"("VME IP Address") -> ()
      n57 = call "ReadQcurve.vi"() -> ("Array"=w83:dbl[])  [unwired: 2 in]
      n58 = Get Date/Time In Seconds() -> (seconds since 1Jan1904=w98:timestamp)
      n59 = To Double Precision Float(number=w98) -> (double precision float=w84:dbl)
      n60 = for {
        N: w97 -> [_]
        tunnel: [w247] -> w100 mode=indexing
        tunnel: w92 -> [w216]
        tunnel: w95 -> [w191]
        tunnel: w94 -> [w203]
        tunnel: w93 -> [w190]
        tunnel: "R&S GPIB Addr (28)" -> [w244]
        tunnel: w96 -> [w243]
        tunnel: w84 -> [w139]
        tunnel: w83 -> [w236]
        tunnel: [w206] -> w86
        tunnel: w76 -> [w169]
        tunnel: w75 -> [w168]
        shift-right: [w161] -> _
        shift-left: w74 -> [w160]
        shift-left: w74 -> [w151]
        shift-left: w74 -> [w159]
        shift-left: w74 -> [w158]
        shift-left: w74 -> [w157]
        shift-left: w74 -> [w156]
        shift-left: w74 -> [w155]
        shift-left: w74 -> [w154]
        shift-left: w74 -> [w153]
        shift-left: w74 -> [w152]
        tunnel: w71 -> [w143]
        tunnel: w70 -> [w142]
        i -> [w149]
        stop <- w141 stop-if-true
        (unwired) 1
        w196 = TRUE
        w211 = 4.9  # Vmax-0.1
        # "Amplify TEQ signal\nfor display"
        # "Adjust tune"
        # "Average signal or noise"
        # "Check voltage limits"
        # "Ave"
        # "Max Pedestal"
        # "Gain sel"
        # "F=real Q"
        # "Real Qcurve\nor quadratic"
        # "+-5V"
        # "Change data plot color if bad"
        # "Max IF offset (V)"
        # "Fmax"
        # "Fmax"
        # "Time"
        # "Vmin"
        # "Raw data"
        # "Corrected Data"
        # "Fcen"
        # "delta F"
        # "# steps"
        # "ADC range"
        # "sweep #"
        # "Set D/A converters, collect data, step frequency upwards, repeat until end of span"
        # "Calculates Q curve"
        # "Removes baseline drift"
        # "Bad voltage or pedestal?"
        # "# steps"
        # "Calculate Fstart"
        # "delta F step"
        n61 = Equal To 0?(x=w149) -> (x = 0?=w249:bool)
        n62 = Divide(x=w203, y=sgl 2.0) -> (x/y=w253:dbl)
        n63 = Subtract(x=w191, y=w253) -> (x-y=w194:dbl)
        n64 = local read "Tune?"() -> (w120:bool)
        n65 = call "Tune.vi"("Init Phase V"=w142, "Init Tune V"=w143, "Tune"=w120) -> ()  [unwired: 9 in]
        n66 = Multiply(x=500.0, y=w203) -> (x*y=w202:dbl)
        n67 = case shown="True" w249 {
          tunnel: w191 -> [_ w300]
          tunnel: w202 -> [_ w301]
          tunnel: [FALSE TRUE] -> w248
          tunnel: w244 -> [_ w297]
          tunnel: w243 -> [_ w296]
          frame False {
            # "Keep current sweep settings"
          }
          frame True {
            # "VME\nReset?"
            # "First sweep"
            # "SETUP RF LEVEL,  FREQUENCY SCAN\nand TURN RF ON. RESET VONTROLLER"
            n68 = case shown="True" FALSE {
              frame False {
              }
              frame True {
                n69 = call "TCPclient.vi"() -> ("Telnet error"=→"Telnet error out":errorcluster)  [unwired: 4 in, 3 out]
              }
            }
            n70 = call "NMRFMsweep.vi"("Center Freq (MHz)"=w300, "Freq Span (kHz)"=w301, "RF Level (dBm)"=w296, "Program"=TRUE, "GPIB Addr (28)"=w297) -> ("error out"=→"SMT error out":errorcluster)  [unwired: 2 in]
          }
        }
        n71 = Add(x=w194, y=w203) -> (x+y=w240:dbl)
        n72 = global read "Global 2.vi" "Subtract Q curve"() -> (w228:bool)
        n73 = global read "Global 2.vi" "Amp of Q curve"() -> (w229:dbl)
        n74 = Select(t=w229, s=w228, f=0.0) -> (s? t:f=w233:dbl)
        n75 = Multiply(x=w236, y=w233) -> (x*y=w235:dbl[])
        n76 = Divide(x=w203, y=w190) -> (x/y=w255:dbl)
        n77 = global read "Global 2.vi" "Invert Polarity"() -> (w177:bool)
        n78 = global read "Global 2.vi" "Gain"() -> (w182:enum16{"LOW", "HI", "MAX"})
        n79 = global read "Global 2.vi" "IFoffset (V)"() -> (w205:dbl)
        n80 = global read "Global 2.vi" "Tune  (V)"() -> (w230:dbl)
        n81 = To Word Integer(number=w255) -> (16bit integer=w252:i16)
        n82 = To Double Precision Float(number=w182) -> (double precision float=w181:dbl)
        n83 = call "Gainsel.vi"("Gain"=w182) -> ("LO"=w208:bool, "MAX"=w207:bool)  [unwired: 1 out]
        n84 = Increment(x=w252) -> (x+1=w150:i16)
        n85 = for {
          N: w150 -> [_]
          tunnel: w160 -> [w265] mode=indexing
          tunnel: w159 -> [w273] mode=indexing
          tunnel: w158 -> [w272] mode=indexing
          tunnel: w157 -> [w271] mode=indexing
          tunnel: w156 -> [w270] mode=indexing
          tunnel: w155 -> [w269] mode=indexing
          tunnel: w154 -> [w268] mode=indexing
          tunnel: w153 -> [w267] mode=indexing
          tunnel: w152 -> [w266] mode=indexing
          tunnel: w151 -> [w274] mode=indexing
          tunnel: [w262] -> w148 mode=indexing
          # "Running sum of 10 sweeps"
          n86 = Compound Arithmetic op=ADD(w265, w274, w273, w272, w271, w270, w269, w268, w267, w266) -> (w263:dbl)
          n87 = Divide(x=w263, y=10) -> (x/y=w262:dbl)
        }
        n88 = Boolean To (0,1)(Boolean=w177) -> (0, 1=w178:i16)
        n89 = Increment(x=w149) -> (x+1=w214:i32)
        "Sweep #" <- w214
        n90 = To Double Precision Float(number=w150) -> (double precision float=w189:dbl)
        n91 = To Double Precision Float(number=w178) -> (double precision float=w176:dbl)
        n92 = stacked-sequence {
          tunnel: [_ w322] -> w192
          tunnel: [_ w326] -> w180
          tunnel: w150 -> [_ w320]
          tunnel: w205 -> [_ w317]
          tunnel: w208 -> [_ w324]
          tunnel: w248 -> [w303 _]
          tunnel: w230 -> [_ w318]
          tunnel: [_ w311] -> w187
          tunnel: [_ w310] -> w133
          tunnel: [_ w318] -> w186
          tunnel: [_ w317] -> w185
          tunnel: [_ w316] -> _
          tunnel: w207 -> [_ w316]
          tunnel: [_ w309] -> w179
          tunnel: w177 -> [_ w308]
          tunnel: [_ w305] -> w175
          frame #0 {
            # "Add code for atten and RF switch here"
            # "Wait for RS SMT frequency to settle"
            n93 = global write "Global 2.vi" "1st Sweep"(w303) -> ()
            n94 = Wait (ms)(milliseconds to wait=10) -> ()  [unwired: 1 out]
            "1st Sweep" <- w303
          }
          frame #1 {
            # "+3.3V"
            # "Offset"
            # "Tune"
            # "Stand dev."
            # "ADCval"
            # "ACQUIRE SINGLE CHANNEL DATA\nCALCULATE MEAN AND ERROR\nSETUP FOR NEG IF VOLTAGE"
            # "# of freq steps"
            n95 = global read "Global 2.vi" "IF / LOG Det"() -> (w307:bool)
            n96 = Boolean To (0,1)(Boolean=w307) -> (0, 1=w306:i16)
            n97 = case shown="False" w307 {
              tunnel: w324 -> [w331 w332]
              tunnel: [w328 w333] -> w321
              frame False {
                n98 = Select "ADC Chan"(t=1, s=w331, f=0) -> (s? t:f=w328:i32)
              }
              frame True {
                n99 = Select "ADC Chan"(t=2, s=w332, f=3) -> (s? t:f=w333:i32)
              }
            }
            n100 = To Double Precision Float(number=w306) -> (double precision float=w305:dbl)
            n101 = global read "Global 2.vi" "# Sample/step"() -> (w313:i32)
            n102 = global read "Global 2.vi" "Tank RF"() -> (w314:bool)
            n103 = global read "Global 2.vi" "IF Atten (dB)"() -> (w312:i8)
            n104 = global read "Global 2.vi" "Logoffset (V)"() -> (w315:dbl)
            n105 = Not(x=w314) -> (.not. x?=w319:bool)
            n106 = global read "Global 2.vi" "Phase (V)"() -> (w309:dbl)
            n107 = call "Netburner_cntlTCP.vi"("Phase Volt"=w309, "Tune Volt"=w318, "# Data"=w313, "IF Atten (dB)"=w312, "NMR ADC"=w321, "Hi Gain"=w316, "Tank RF"=w319, "LogOff Volt"=w315, "IFOff Volt"=w317, "# f steps"=w320) -> ("Temp (C)"=w311:dbl, "ADC value"=w323:dbl[], "ADC Std Dev"=w322:dbl, "Volts"=w310:dbl)  [unwired: 2 out]
            "Temp (C)" <- w311
            "+3.3V supply" <- w310
            n108 = global write "Global 2.vi" "+3V supply"(w310) -> ()
            n109 = global write "Global 2.vi" "Temp (C)"(w311) -> ()
            n110 = Negate(x=w323) -> (-x=w325:dbl[])
            n111 = Wait (ms)(milliseconds to wait=1) -> ()  [unwired: 1 out]
            n112 = Select(t=w325, s=w308, f=w323) -> (s? t:f=w326:dbl[])
          }
        }
        n113 = global write "Global 2.vi" "Sweep #"(w214) -> ()
        n114 = call "Qcorrect.vi"("Subtract Q curve"=w228, "Nstep"=w150, "Max Gain"=w207, "Amp of Q curve"=w229, "Step Width (MHz)"=w190, "Center Freq (MHz)"=w191) -> ("Start"=w250:i32, "Array"=w251:dbl[])
        n115 = global read "Global 2.vi" "Real/Quad Q curve"() -> (w227:bool)
        n116 = To Double Precision Float(number=w214) -> (double precision float=w188:dbl)
        n117 = Array Subset "Array Subset"(array=w251, index=w250, length=w150) -> (w237:dbl[])
        n118 = property on="Property Node" class="VI"(reference=w169, error in=w168) -> ("Exec.State"=w171:T2)  [unwired: 2 out]
        n119 = global read "Global 2.vi" "AutoTune"() -> (w225:bool)
        n120 = Select(t=w237, s=w227, f=w235) -> (s? t:f=w163:dbl[])
        n121 = Not(x=w225) -> (.not. x?=w238:bool)
        n122 = Equal?(x=2, y=w171) -> (x = y?=→"He readback":bool)
        n123 = Not(x="Stop Run") -> (.not. x?=w141:bool)
        n124 = Greater?(x=w205, y=7.5) -> (0:w241:bool)
        n125 = Not(x=w241) -> (.not. x?=w221:bool)
        "RF level OK" <- w221
        n126 = global write "Global 2.vi" "RF OK"(w221) -> ()
        n127 = case shown="True" w141 {
          frame False {
          }
          frame True {
            n128 = stacked-sequence {
              frame #0 {
                n129 = Wait (ms)(milliseconds to wait=100) -> ()  [unwired: 1 out]
              }
              frame #1 {
                n130 = Stop() -> ()  [unwired: 1 in]
              }
            }
          }
        }
        n131 = global read "Global 2.vi" "Amp of Q curve"() -> (w183:dbl)
        n132 = To Double Precision Float(number=w214) -> (double precision float=w209:dbl)
        n133 = global read "Global 2.vi" "RemovePed"() -> (w226:bool)
        n134 = Equal To 0?(x=w149) -> (x = 0?=w213:bool)
        n135 = call "RemoveQandP.vi"("Subtract Ped?"=w226, "Qcurve"=w163, "Raw data"=w180) -> ("Ped L-R"=w114:dbl, "Corrected data"=w199:dbl[], "Ped Offfset"=w121:dbl)
        "Pedestal (V)" <- w121
        n136 = Multiply(x=w121, y=10.0) -> (x*y=w231:dbl)
        n137 = call "Autozero.vi"("Vmin (V)"=w231, "IFoffset (V)"=w205, "Enable"=w238, "Max Gain"=w207) -> ()
        n138 = global write "Global 2.vi" "Pedestal Offset"(w121) -> ()
        n139 = global read "Global 2.vi" "Gauss Fit"() -> (w224:bool)
        n140 = global write "Global 2.vi" "Sample RMS (V)"(w192) -> ()
        n141 = Get Date/Time In Seconds() -> (seconds since 1Jan1904=w147:timestamp)
        n142 = Subtract(x=w133, y=3.3) -> (x-y=w135:dbl)
        n143 = global write "Global 2.vi" "Temperature (C)"(w187) -> ()
        n144 = Array Max & Min "Array Max"(array=w199) -> (max value=w184:dbl)  [unwired: 3 out]
        n145 = Absolute Value(x=w135) -> (abs(x)=w134:dbl)
        n146 = call-poly <vilib>:"Power Spectrum.vi"("X"=w180) -> ("Power Spectrum"=w204:dbl[])  [unwired: 1 out]
        n147 = Less?(x=w134, y=0.1) -> (x < y?=→"+3.3V OK":bool)
        n148 = global read "Global 2.vi" "Calib Constant"() -> (w138:dbl)
        n149 = Absolute Value ("Abs Value")(x=w114) -> (abs(x)=w245:dbl)
        n150 = Negate(x=w114) -> (-x=w119:dbl)
        "Pedestal Diff (V)" <- w119
        n151 = call "FitData.vi"("Fit?"=w224, "Fmax"=w240, "Fmin"=w194, "Yarray"=w199) -> ("Peak Area (mV-MHz)"=w104:dbl, "Center Freq (MHz)"=w107:dbl, "NMR Graph + Fit"=w220:cluster{cluster{dbl, "Numeric":dbl}[]}[])  [unwired: 2 out]
        n152 = Build Array (concatenate) "Header + Data"(w191, w190, w189, w188, w187, w133, w186, w185, w179, w104, w183, w138, w181, w176, w175, w180) -> (w140:dbl[])
        n153 = global write "Global 2.vi" "NMR Graph + Fit"(w220) -> ()
        n154 = Square Root(x=w204) -> (sqrt(x)=w200:dbl[])
        "FFT Vrms" <- w200
        n155 = global read "Global 2.vi" "Subtract Q curve"() -> (w109:bool)
        n156 = call "SaveTune.vi"("Array"=w140, "Save Data to File"="Save Tune", "Ext time (sec)"=w139) -> ()  [unwired: 1 out]
        n157 = global write "Global 2.vi" "Pedestal Difference"(w119) -> ()
        n158 = global write "Global 2.vi" "Pedestal Diff (V)"(w119) -> ()
        n159 = Select(t=w180, s=w196, f=w200) -> (s? t:f=w161:dbl[])
        n160 = Format Date/Time String(time format string (%c)="%c", seconds (now)=w147) -> (date/time string=→"Date / Time":string)  [unwired: 1 in]
        n161 = call "SaveData.vi"("Quad sub area"=w104, "Ext time (sec)"=w139, "Array"=w140) -> ("Frequency"=w108:dbl, "Area"=w137:dbl, "ADC value"=w129:dbl[])  [unwired: 1 out]
        n162 = feedback #2 "Feedback Node"() -> (w212:dbl[])  [unwired: 1 in]
        n163 = case shown="False" w213 {
          tunnel: w161 -> [w284 w286]
          tunnel: [w283 w286] -> w210
          tunnel: w212 -> [w285 _]
          frame False {
            # "Sum sweeps"
            n164 = Add(x=w285, y=w284) -> (x+y=w283:dbl[])
          }
          frame True {
            # "Initialize"
          }
        }
        n165 = feedback-in #2(w210) -> ()
        n166 = Divide(x=w210, y=w209) -> (x/y=w162:dbl[])
        n167 = Multiply(x=w138, y=w184) -> (x*y=w113:dbl)
        "Peak amp (mV)" <- w113
        n168 = Select(t=0.1, s=w207, f=0.1) -> (s? t:f=w215:dbl)
        n169 = Multiply(x=w137, y=w138) -> (x*y=w112:dbl)
        n170 = Multiply(x=w104, y=w138) -> (x*y=w110:dbl)
        n171 = Not(x=w109) -> (.not. x?=w106:bool)
        n172 = Greater?(x=w245, y=w215) -> (0:w217:bool)
        n173 = call "ADCok.vi"("PedOK"=w217, "Array"=w180, "Vmax-1/2"=w211) -> ("ADC voltages OK"=w223:bool, "Allok"=w239:bool)  [unwired: 1 out]
        "ADC volts OK" <- w223
        n174 = global read "Global - Pressure & Flow.vi" "Task3 Temperature"() -> (→"He temp (K)":dbl)
        n175 = global read "Global - Pressure & Flow.vi" "Task3 Pressure"() -> (→"He press (torr)":dbl)
        n176 = And(x=w239, y=w216) -> (x .and. y?=w246:bool)
        n177 = case shown="False" w239 {
          frame False {
            # "All OK"
            n178 = property on="Raw NMR Graph / Ave" class="WFGraph (strict)"("Active Plot"=0, "Plot.Plot Color"=u32 13145856) -> ()  [unwired: 2 in, 2 out]
          }
          frame True {
            # "Bad data"
            n179 = property on="Raw NMR Graph / Ave" class="WFGraph (strict)"("Active Plot"=0, "Plot.Plot Color"=u32 16711680) -> ()  [unwired: 2 in, 2 out]
          }
        }
        n180 = Not(x=w217) -> (.not. x?=w222:bool)
        "Pedestal volts OK" <- w222
        n181 = Select(t=w112, s=w106, f=w110) -> (s? t:f=w111:dbl)
        "Polarization %" <- w111
        "Polarization" <- w111
        n182 = global read "Global 2.vi" "Subtract Q curve"() -> (w164:bool)
        n183 = Select(t=w194, s=w196, f=0.0) -> (s? t:f=w193:dbl)
        n184 = Select(t=w190, s=w196, f=1.0) -> (s? t:f=w197:dbl)
        n185 = global write "Global 2.vi" "Pedestal OK"(w222) -> ()
        n186 = Select(t=w108, s=w106, f=w107) -> (s? t:f=w105:dbl)
        "Peak center (MHz)" <- w105
        n187 = global write "Global 2.vi" "ADC volts OK"(w223) -> ()
        n188 = case shown="True" w246 {
          tunnel: [w291 -99.0] -> w247
          tunnel: w111 -> [w291 _]
          frame False {
            # "Data OK"
          }
          frame True {
            # "flag it bad"
          }
        }
        n189 = global write "Global 2.vi" "Peak center (MHz)"(w105) -> ()
        n190 = global write "Global 2.vi" "Peak Height"(w111) -> ()
        n191 = global read "Global 2.vi" "AutoFreq"() -> (w115:bool)
        n192 = local read "Tune?"() -> (w118:bool)
        n193 = global write "Global 2.vi" "Peak amp (V)"(w113) -> ()
        n194 = global read "Global 2.vi" "Measurement"() -> (w127:enum16{"TEQ", "POL", "QCV"})
        n195 = global write "Global 2.vi" "Peak area (mV-MHz)"(w111) -> ()
        n196 = Not(x=w118) -> (.not. x?=w116:bool)
        n197 = And(x=w115, y=w116) -> (x .and. y?=w117:bool)
        n198 = Not Equal?(x=w127, y=1) -> (x != y?=w125:bool)
        n199 = case shown="True" w117 {
          tunnel: w114 -> [_ w256]
          frame False {
          }
          frame True {
            n200 = global read "Global 2.vi" "Tune  (V)"() -> (w258:dbl)
            n201 = Divide(x=w256, y=50.0) -> (x/y=w259:dbl)
            n202 = Subtract(x=w258, y=w259) -> (x-y=w257:dbl)
            n203 = global write "Global 2.vi" "Tune  (V)"(w257) -> ()
          }
        }
        n204 = Select(t=10.0, s=w125, f=1.0) -> (s? t:f=w122:dbl)
        n205 = Multiply(x=w129, y=w122) -> (x*y=w128:dbl[])
        n206 = case shown="True" w164 {
          tunnel: w161 -> [w278 w282]
          tunnel: [w277 w281] -> w165
          tunnel: w163 -> [_ w280]
          tunnel: w148 -> [w276 w279]
          tunnel: w128 -> [w275 _]
          frame False {
            n207 = Build Array(w278, w276, w275) -> (w277:dbl[][])
          }
          frame True {
            n208 = Build Array(w282, w279, w280) -> (w281:dbl[][])
          }
        }
        n209 = Bundle(w193, "Step Width (MHz)"=w197, w165) -> (→"Raw NMR Graph / Ave":cluster{dbl, "Step Width (MHz)":dbl, dbl[][]})  [unwired: 1 in]
        n210 = global read "Global 2.vi" "Fit OK"() -> (→"Qsub OK":bool)
        n211 = Build Array (concatenate) "Build Array"(w193, w197, w162) -> (w206:dbl[])
      }
      n212 = call "DataQA.vi"("Quality cuts"=w92, "Data In"=w100) -> ("Data Out"=w99:dbl[])
      n213 = global read "Global 2.vi" "Save Data to File"() -> (w85:bool)
      n214 = call <vilib>:"Std Deviation and Variance.vi"("X"=w99) -> ("mean"=w90:dbl, "standard deviation"=w80:dbl)  [unwired: 1 in, 1 out]
      "Polarization %" <- w90
      n215 = Multiply(x=w80, y=1.0) -> (x*y=→"Pol sdev":dbl)
      n216 = call "PeakHisto.vi"("Data Out"=w99) -> ("XY Graph"=w88:cluster{"Y":dbl[], "Y":dbl[]}[])
      "Peak Height Distribution" <- w88
      n217 = global write "Global 2.vi" "Peak Height Distribution"(w88) -> ()
      n218 = global write "Global 2.vi" "Peak mean (V)"(w90) -> ()
      n219 = call "SaveDataAve.vi"("Array"=w86, "Save Data to File"=w85) -> ()  [unwired: 1 in, 1 out]
      n220 = Array Size(array=w99) -> (size(s)=w89:i32)
      "# Good Spectra" <- w89
      n221 = global write "Global 2.vi" "# Good Spectra"(w89) -> ()
      n222 = Divide(x=w90, y=w80) -> (x/y=w91:dbl)
      "S/N" <- w91
      n223 = global write "Global 2.vi" "S/N"(w91) -> ()
    }
    frame #2 {
      n224 = property on="Property Node" class="VI"(reference=w337, error in=w336) -> (reference out=w339:refnum<vi>, error out=w338:errorcluster, "Exec.State"=w341:T2)
      n225 = Equal?(x=2, y=w341) -> (x = y?=w340:bool)
      n226 = case shown="True" w340 {
        tunnel: w339 -> [_ w348]
        tunnel: w338 -> [_ w347]
        frame False {
        }
        frame True {
          # "Stop MKS routine and close panel if running"
          # "Add simple error handling\nfor VI operations"
          n227 = invoke on="Invoke Node" class="VI" method="Abort VI"(reference=w348, error in=w347) -> (reference out=w345:refnum<vi>, error out=w344:errorcluster)  [unwired: 1 in, 1 out]
          n228 = property on="Property Node" class="VI"(reference=w345, error in=w344, "Front Panel Window:Open"=FALSE) -> (error out=w343:errorcluster)  [unwired: 1 out]
          n229 = call <vilib>:"Simple Error Handler.vi"("type of dialog (OK msg:1)"=1, "error in (no error)"=w343) -> ()  [unwired: 3 in, 5 out]
        }
      }
    }
  }
